vi "Recompile_specified_files.vi"() -> (1 "Saved Vis paths Out":string[](array[string]))   [LabVIEW 2020]
uses:
  Anemometry Sub Vis/Globals/Constants_global.vi
panel:
  out "Progress":i32(slide) scale=0.0..1935.0
  in  "stop":bool
  out "Time taken for convertion (min)":dbl format="%.2f"
  out "Broken vi's":string[](array[string])
  out "Current top level":path
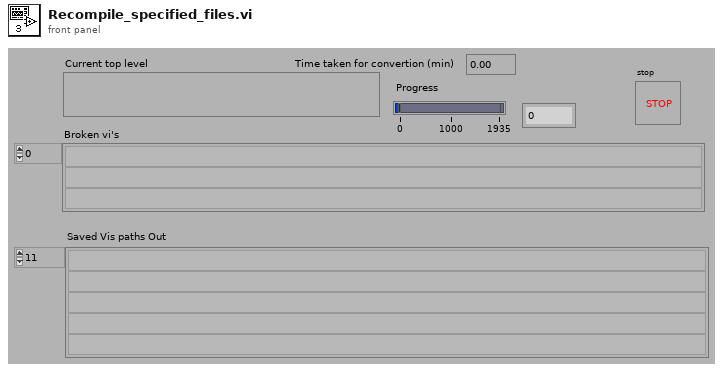
[diagram p1: front panel]
types:
  T1 = enum32{"Bad", "Idle", "Run top level", "Running"}
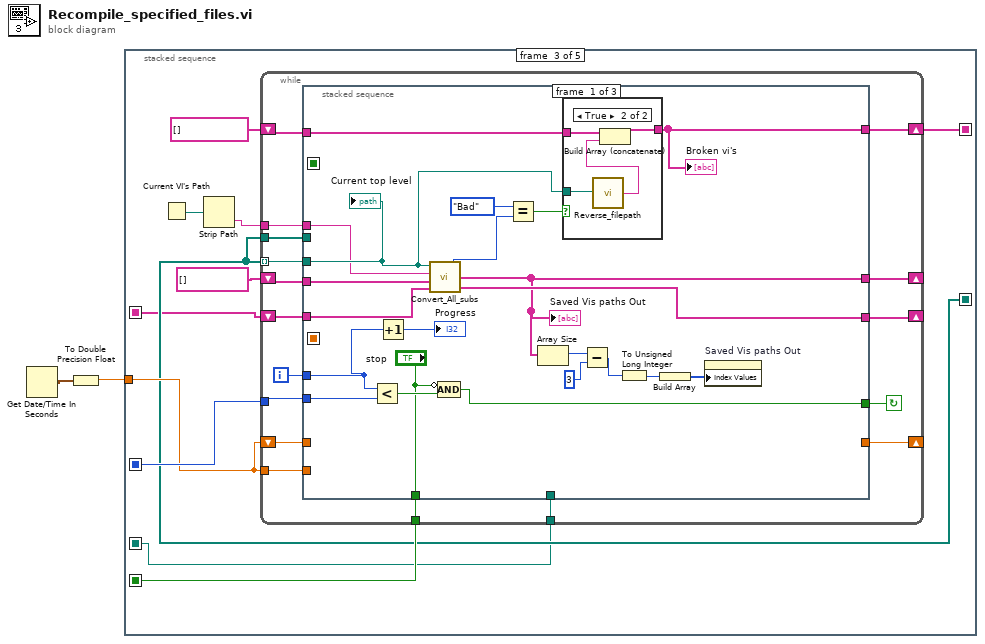
[diagram p0: block diagram]
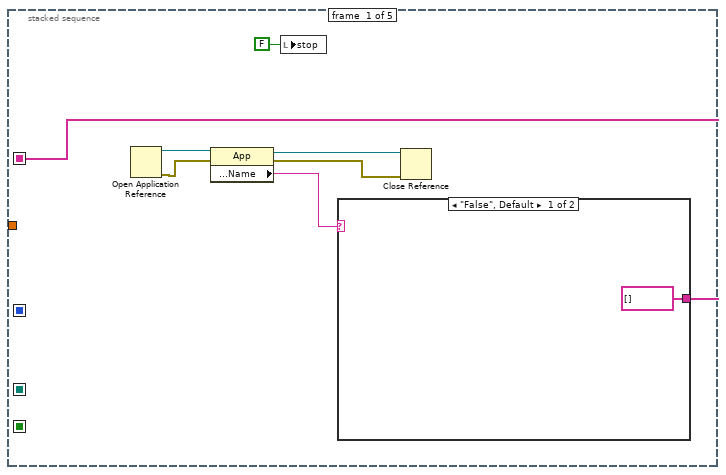
[diagram p2: hidden frame]
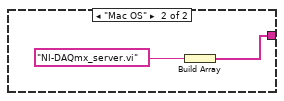
[diagram p3: hidden frame]
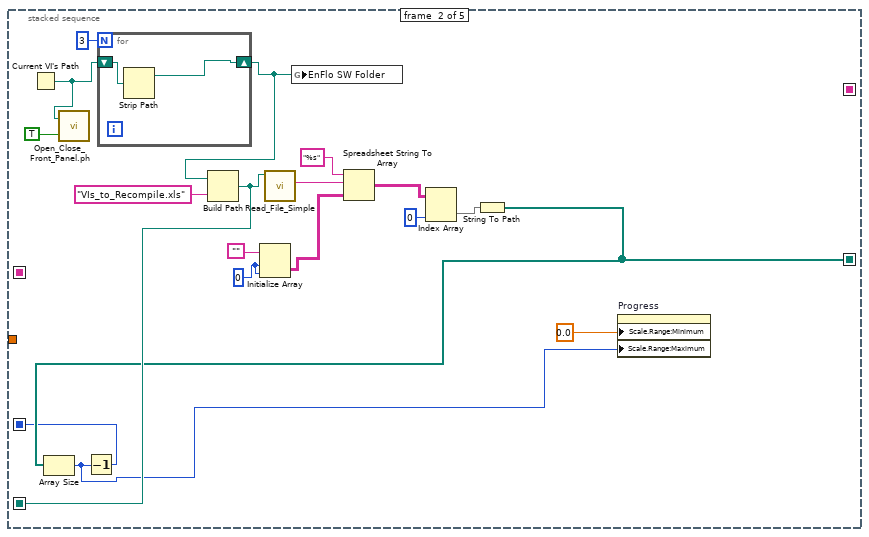
[diagram p4: hidden frame]
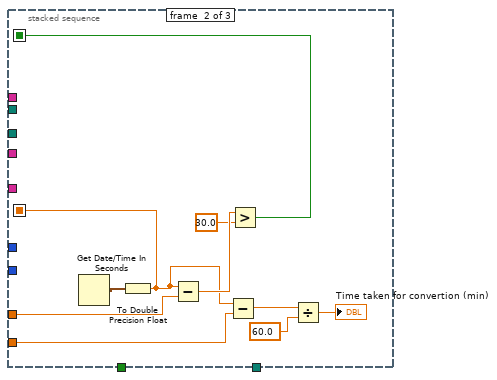
[diagram p6: hidden frame]
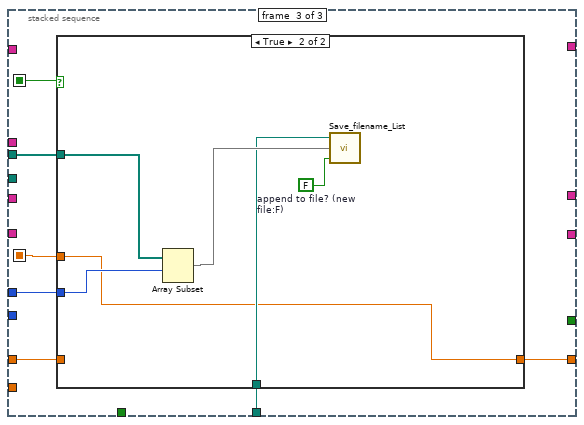
[diagram p7: hidden frame]
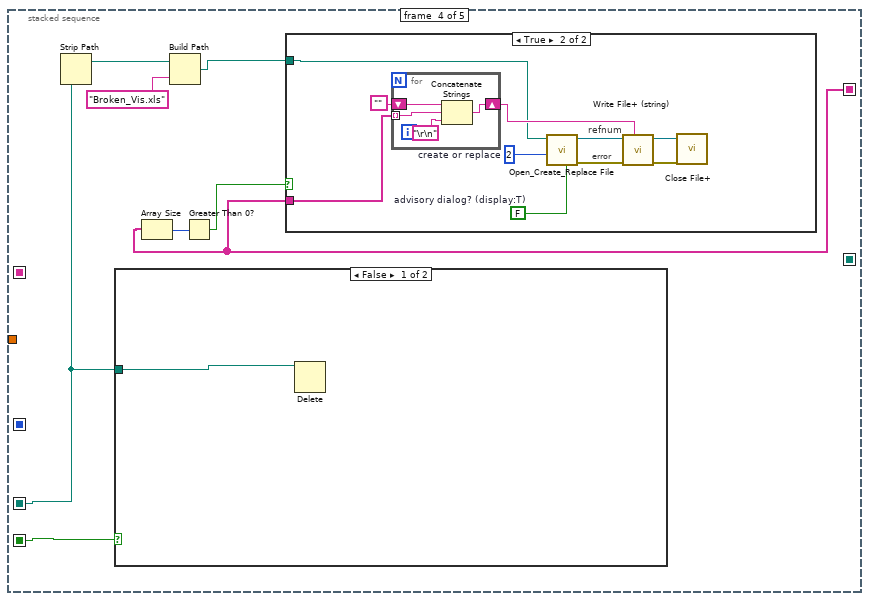
[diagram p9: hidden frame]
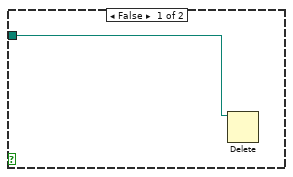
[diagram p10: hidden frame]
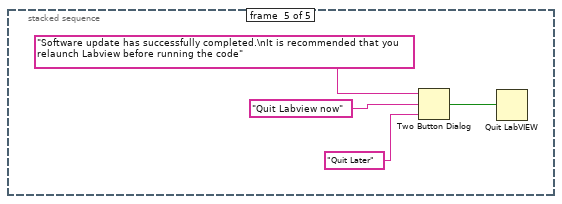
[diagram p12: hidden frame]
diagram:
  n1 = Get Date/Time In Seconds() -> (seconds since 1Jan1904=w1:timestamp)
  n2 = To Double Precision Float(number=w1) -> (double precision float=w2:dbl)
  n3 = stacked-sequence {
    seq-local: [_ w15 _ _ _] -> [_ _ w36 _ _]
    seq-local: [_ _ w41 _ _] -> [_ _ _ w119 _]
    seq-local: [_ w16 _ _ _] -> [_ _ w35 w118 _]
    seq-local: [_ w14 _ _ _] -> [_ _ w38 _ _]
    seq-local: [_ _ w34 _ _] -> [_ _ _ w113 _]
    seq-local: [w3 _ _ _ _] -> [_ _ w33 _ _]
    tunnel: w2 -> [_ _ w37 _ _]
    frame #0 {
      n4 = Open Application Reference() -> (0:w8:errorcluster, 3:w7:refnum<vi>)  [unwired: 1 in, 3 out]
      n5 = property class="App"(reference=w7, error in=w8) -> (reference out=w6:refnum<vi>, error out=w5:errorcluster, "Operating System:Name"=w4:string)
      n6 = local write "stop"(FALSE ("stop")) -> ()
      n7 = case shown="\"False\", Default" w4 {
        tunnel: [string[] [] w11] -> w3
        frame "False", Default {
        }
        frame "Mac OS" {
          n8 = Build Array("NI-DAQmx_server.vi") -> (w11:string[])
        }
      }
      n9 = Close Reference(reference=w6, error in (no error)=w5) -> ()  [unwired: 1 out]
    }
    frame #1 {
      w27 = 0 ("Dimension Size")
      n10 = Current VI's Path() -> (path=w18:path)
      n11 = call "Open_Close_Front_Panel.ph.vi"("openWindow (T)"=TRUE ("Front Panel Window:Open"), "VI path"=w18) -> ()  [unwired: 2 out]
      n12 = for {
        N: 3 -> [_]
        shift-right: [w31] -> w20
        shift-left: w18 -> [w32]
        n13 = Strip Path(path=w32) -> (stripped path=w31:path)  [unwired: 1 out]
      }
      n14 = Build Path(base path=w20, name or relative path="VIs_to_Recompile.xls") -> (appended path=w16:path)
      n15 = Initialize Array("", w27, w27) -> (w25:string[][])
      n16 = call "Read_File_Simple.vi"("Filename"=w16) -> ("string"=w28:string)  [unwired: 2 in, 7 out]
      n17 = global write "Constants_global.vi" "EnFlo SW Folder"(w20) -> ()
      n18 = Spreadsheet String To Array(format string="%s", spreadsheet string=w28, array type (2D Dbl)=w25) -> (array=w23:string[][])  [unwired: 1 out]
      n19 = Index Array(array=w23, index (col)=0 ("disabled index (col)")) -> (element=w22:string[])  [unwired: 1 in]
      n20 = String To Path(string=w22) -> (path=w15:path[])
      n21 = Array Size(array=w15) -> (size(s)=w13:i32)
      n22 = Decrement(x=w13) -> (x-1=w14:i32)
      n23 = property on="Progress" class="Slide (strict)"("Scale.Range:Minimum"=0.0 ("Data Range:Minimum"), "Scale.Range:Maximum"=w13) -> ()  [unwired: 2 in, 2 out]
    }
    frame #2 {
      n24 = Current VI's Path() -> (path=w40:path)
      n25 = Strip Path(path=w40) -> (name=w39:string)  [unwired: 1 out]
      n26 = while {
        tunnel: w38 -> [w53]
        shift-left: string[] [] ("Saved Vis paths Out") -> [w57]
        shift-right: [w54] -> _
        shift-left: string[] [] -> [w56]
        shift-right: [w55] -> w34
        shift-left: w33 -> [w60]
        shift-right: [w59] -> _
        tunnel: w36 -> [w58] mode=indexing
        tunnel: [w51] -> w41
        tunnel: w39 -> [w50]
        tunnel: w37 -> [w48]
        shift-right: [w44] -> _
        shift-left: w37 -> [w47]
        tunnel: w36 -> [w46]
        tunnel: w35 -> [w45]
        i -> [w49]
        stop <- w52 continue-if-true
        n27 = stacked-sequence {
          seq-local: [_ w89 _] -> [_ _ w101]
          seq-local: [_ w88 _] -> [_ _ w100]
          tunnel: w60 -> [w82 _ _]
          tunnel: [w81 _ _] -> w59
          tunnel: w58 -> [w80 _ _]
          tunnel: w57 -> [w76 _ _]
          tunnel: w56 -> [w75 _ _]
          tunnel: [w74 _ _] -> w55
          tunnel: [w73 _ _] -> w54
          tunnel: w53 -> [w67 _ _]
          tunnel: [w65 _ _] -> w52
          tunnel: ["stop" _ _] -> w51
          tunnel: w50 -> [w63 _ _]
          tunnel: w49 -> [w62 _ w104]
          tunnel: w48 -> [_ w92 _]
          tunnel: w47 -> [_ w96 w98]
          tunnel: w46 -> [_ _ w103]
          tunnel: w45 -> [_ _ w102]
          tunnel: [_ _ w99] -> w44
          frame #0 {
            n28 = Less?(x=w62, y=w67) -> (x < y?=w66:bool)
            n29 = Increment(x=w62) -> (x+1=→"Progress":i32)
            n30 = call "Convert_All_subs.vi"("Shift in"=w82, "Saved Vis paths in"=w76, "Top level VI Name"=w63, "VI path"=w80) -> ("Shift out"=w81:string[], "Saved Vis paths Out"=w73:string[], "Exec.State"=w78:T1)
            "Saved Vis paths Out" <- w73
            n31 = Compound Arithmetic op=AND(invert "stop", w66) -> (w65:bool)
            n32 = Equal?(x=T1."Bad" ("Exec.State"), y=w78) -> (x = y?=w77:bool)
            n33 = Array Size(array=w73) -> (size(s)=w72:i32)
            n34 = case shown="True" w77 {
              tunnel: w80 -> [_ w85]
              tunnel: w75 -> [w83 w87]
              tunnel: [w83 w86] -> w74
              frame False {
              }
              frame True {
                n35 = call "Reverse_filepath.vi"("Filename"=w85) -> ("Reversed Filepath"=w84:string)
                n36 = Build Array (concatenate)(w87, w84) -> (w86:string[])
              }
            }
            "Broken vi's" <- w74
            n37 = Subtract(x=w72, y=3) -> (x-y=w70:i32)
            n38 = To Unsigned Long Integer(number=w70) -> (unsigned 32bit integer=w69:u32)
            n39 = Build Array(w69) -> (w68:u32[])
            n40 = property on="Saved Vis paths Out" class="Arr (strict)"("Index Values"=w68) -> ()  [unwired: 2 in, 2 out]
            "Current top level" <- w80
          }
          frame #1 {
            n41 = Get Date/Time In Seconds() -> (seconds since 1Jan1904=w97:timestamp)
            n42 = To Double Precision Float(number=w97) -> (double precision float=w88:dbl)
            n43 = Subtract(x=w88, y=w96) -> (x-y=w91:dbl)
            n44 = Subtract(x=w88, y=w92) -> (x-y=w94:dbl)
            n45 = Greater?(x=w91, y=30.0) -> (0:w89:bool)
            n46 = Divide(x=w94, y=60.0) -> (x/y=→"Time taken for convertion (min)":dbl)
          }
          frame #2 {
            n47 = case shown="True" w101 {
              tunnel: w104 -> [_ w111]
              tunnel: w103 -> [_ w110]
              tunnel: w102 -> [_ w108]
              tunnel: w100 -> [_ w107]
              tunnel: [w105 w107] -> w99
              tunnel: w98 -> [w105 _]
              frame False {
              }
              frame True {
                w106 = FALSE  # append to file? (new file:F)
                n48 = Array Subset(array=w110, index=w111) -> (w109:path[])  [unwired: 1 in]
                n49 = call "Save_filename_List.vi"("append to file? (new file:F)"=w106, "Filename to save"=w109, "file path (dialog if empty)"=w108) -> ()  [unwired: 1 out]
              }
            }
          }
        }
      }
    }
    frame #3 {
      n50 = Strip Path(path=w118) -> (stripped path=w117:path)  [unwired: 1 out]
      n51 = case shown="False" w119 {
        tunnel: w118 -> [w135 _]
        frame False {
          n52 = Delete(path (use dialog)=w135) -> ()  [unwired: 1 in, 6 out]
        }
        frame True {
        }
      }
      n53 = Array Size(array=w113) -> (size(s)=w114:i32)
      n54 = Build Path(base path=w117, name or relative path="Broken_Vis.xls") -> (appended path=w115:path)
      n55 = Greater Than 0?(x=w114) -> (x > 0?=w112:bool)
      n56 = case shown="True" w112 {
        tunnel: w115 -> [w120 w122]
        tunnel: w113 -> [_ w125]
        frame False {
          n57 = Delete(path (use dialog)=w120) -> ()  [unwired: 1 in, 6 out]
        }
        frame True {
          w121 = FALSE  # advisory dialog? (display:T)
          w126 = i16 2  # create or replace
          # "error"
          # "refnum"
          n58 = for {
            shift-right: [w131] -> w123
            shift-left: "" -> [w134]
            tunnel: w125 -> [w132] mode=indexing
            n59 = Concatenate Strings(w134, w132, "\r\n") -> (w131:string)
          }
          n60 = call <vilib>:"Open_Create_Replace File.vi"("advisory dialog? (display:T)"=w121, "function (open:0)"=w126, "file path"=w122) -> ("error out"=w130:errorcluster, "refnum"=w127:refnum<file>)  [unwired: 4 in, 3 out]
          n61 = call <vilib>:"Write File+ (string).vi"("string"=w123, "error in (no error)"=w130, "refnum"=w127) -> ("error out"=w129:errorcluster, "dup refnum"=w128:refnum<file>)  [unwired: 2 in, 3 out]
          n62 = call <vilib>:"Close File+.vi"("error in (no error)"=w129, "refnum"=w128) -> ()  [unwired: 6 out]
        }
      }
    }
    frame #4 {
      n63 = Two Button Dialog(message="Software update has successfully completed.\nIt is recommended that you relaunch Labview before running the code", 1:"Quit Later" ("F button name (\"Cancel\")"), 2:"Quit Labview now" ("button name (\"OK\")")) -> (T button?=w136:bool)
      n64 = Quit LabVIEW(quit? (T)=w136) -> ()
    }
  }
